vi "Teleop.vi"(10 "Match Info":T1={"Autonomous Elapsed Seconds"=0.0, "TeleOp Elapsed Seconds"=0.0, "Disabled Elapsed Seconds"=0.0, "Visited Autonomous"=FALSE, "Visited TeleOp"=FALSE, "Visited Disabled"=FALSE, "Autonomous Settings"={"Autonomous Style"=enum."Independent", "VI Refnum"=refnum}}, 11 "Call Context":T2) -> ()   [LabVIEW 2013]
doc: "This VI is called for each TeleOp packet received from the DS where the robot is not disabled. It is often used to read from the joysticks and update I/O or to update setpoints for timed control loops. It should complete and return within 20 milliseconds or it may miss DS packets."
uses:
  <vilib>/Rock Robotics/WPI/DriverStation/WPI_DriverStationDerivedRobotMode.ctl
  <vilib>/Rock Robotics/WPI/DriverStation/WPI_DriverStationMatch Info.ctl
  <vilib>/Rock Robotics/WPI/Solenoid/WPI_SolenoidValue.ctl
  Robot Global Data.vi
  <vilib>/Rock Robotics/WPI/Joystick/WPI_JoystickGetSetRefNum.vi
  <vilib>/Rock Robotics/WPI/Solenoid/Deprecated/WPI_SolenoidGetBool.vi
  <vilib>/Rock Robotics/WPI/Solenoid/WPI_SolenoidSetEnum.vi
  <vilib>/Rock Robotics/WPI/RobotDrive/WPI_RobotDriveGetSetRefNum.vi
  Labview/Sub VIs/Sting Pot Value.vi
panel:
  out "Voltage":dbl
  out "Value":bool
  out "Numeric 1":dbl(slide) scale=0.0..100.0
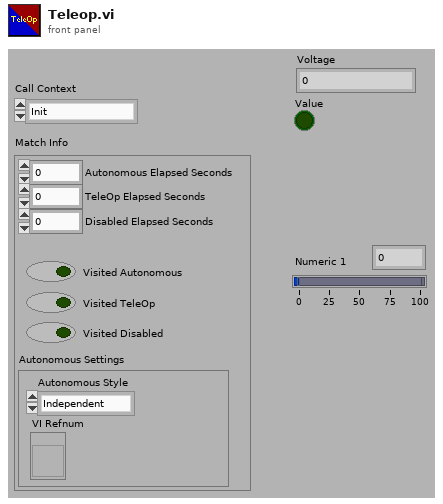
[diagram p1: front panel]
types:
  T1 = typedef "WPI_DriverStationMatch Info.ctl" = cluster{"Autonomous Elapsed Seconds":dbl, "TeleOp Elapsed Seconds":dbl, "Disabled Elapsed Seconds":dbl, "Visited Autonomous":bool, "Visited TeleOp":bool, "Visited Disabled":bool, "Autonomous Settings":cluster{"Autonomous Style":enum16{"Iterative", "Independent"}, "VI Refnum":refnum<vi>}}
  T2 = typedef "WPI_DriverStationDerivedRobotMode.ctl" = enum16{"Init", "Execute", "Stop"}
  T3 = typedef "WPI_JoystickDevRef.ctl" = cluster{"Device":T4}
  T4 = typedef "WPI_JoystickDeviceEnum.ctl" = enum16{"USB 1", "USB 2", "USB 3", "USB 4", "Kinect 1", "Kinect 2"}
  T5 = typedef "WPI_JoystickButtonState.ctl" = cluster{"Button 1":bool, "Button 2":bool, "Button 3":bool, "Button 4":bool, "Button 5":bool, "Button 6":bool, "Button 7":bool, "Button 8":bool, "Button 9":bool, "Button 10":bool, "Button 11":bool, "Button 12":bool}
  T6 = typedef "WPI_MotorControlDeviceRef.ctl" = cluster{"DeviceStatus":errorcluster, "Type":enum16{"PWM", "CAN"}, "PWM":cluster{"Digital Module":T7, "PWM Channel":T8, "DeadBand":T9}, "CAN":cluster{"Device Number":u8, "Control Mode":T10, "Semaphore":T11, "Max Vout":dbl}, "Invert":bool, "TransformRef":T12, "InvTransformRef":T12}
  T7 = typedef "FPGA_TypedefDigitalModule.ctl" = enum16{"Digital Module 1", "Digital Module 2"}
  T8 = typedef "FPGA_DIOPWMChannel.ctl" = enum8{"PWM 1", "PWM 2", "PWM 3", "PWM 4", "PWM 5", "PWM 6", "PWM 7", "PWM 8", "PWM 9", "PWM 10", "Invalid"}
  T9 = typedef "WPI_PWMDeadband.ctl" = cluster{"Name":string, "maxPositivePwm":i32, "minPositivePwm":i32, "centerPwm":i32, "maxNegativePwm":i32, "minNegativePwm":i32, "angularRange":u16}
  T10 = typedef "WPI_CANJaguar_ControlMode.ctl" = enum8{"Percent VBus", "Current", "Speed", "Position", "Voltage"}
  T11 = typedef "Semaphore RefNum" = refnum<k1>
  T12 = typedef "WPI_PWMTransform_ConPane.ctl" = refnum<vi>
  T13 = typedef "WPI_AnalogChannelDevRef.ctl" = cluster{"DevStatus":errorcluster, "Analog Module":T14, "Analog Channel":T15}
  T14 = typedef "FPGA_TypedefAnalogModule.ctl" = enum16{"Analog Module 1", "Analog Module 2"}
  T15 = typedef "FPGA_AIChannel.ctl" = enum8{"AI 1", "AI 2", "AI 3", "AI 4", "AI 5", "AI 6", "AI 7", "AI 8", "Invalid"}
  T16 = cluster{"axis 1 (x)":dbl, "axis 2 (y)":dbl, "axis 3 (throttle)":dbl, "axis 4":dbl, "axis 5":dbl, "axis 6":dbl}
  T17 = typedef "WPI_RobotDriveDevRef.ctl" = cluster{"DevStatus":errorcluster, "Motors[]":T6[], "Square Inputs":bool, "Max Output":dbl, "Isochronous":bool}
  T18 = typedef "WPI_RelayDevRef.ctl" = cluster{"DevStatus":errorcluster, "Relay Channel":T19, "Digital Module":T7, "Relay Direction":T20}
  T19 = typedef "FPGA_DIORelayChannel.ctl" = enum8{"Relay 1", "Relay 2", "Relay 3", "Relay 4", "Relay 5", "Relay 6", "Relay 7", "Relay 8", "Invalid"}
  T20 = typedef "WPI_RelayDirection.ctl" = enum16{"Both directions", "Forward only", "Reverse only"}
  T21 = typedef "WPI_DigitalInputDevRef.ctl" = cluster{"DevStatus":errorcluster, "DIO Channel":T22, "Digital Module":T7}
  T22 = typedef "FPGA_DIOChannel.ctl" = enum8{"DIO 1", "DIO 2", "DIO 3", "DIO 4", "DIO 5", "DIO 6", "DIO 7", "DIO 8", "DIO 9", "DIO 10", "DIO 11", "DIO 12", "DIO 13", "DIO 14", "Invalid"}
  T23 = typedef "WPI_SolenoidValue.ctl" = enum16{"Off", "On", "Forward", "Reverse"}
  T24 = typedef "WPI_SolenoidDevRef.ctl" = cluster{"DevStatus":errorcluster, "Solenoid Module":T25, "Forward Solenoid Channel":T26, "Reverse Solenoid Channel":T26}
  T25 = typedef "FPGA_TypedefSolenoidModule.ctl" = enum16{"Solenoid Module 1", "Solenoid Module 2"}
  T26 = typedef "WPI_SolenoidChannel.ctl" = enum8{"Solenoid 1", "Solenoid 2", "Solenoid 3", "Solenoid 4", "Solenoid 5", "Solenoid 6", "Solenoid 7", "Solenoid 8", "Invalid"}
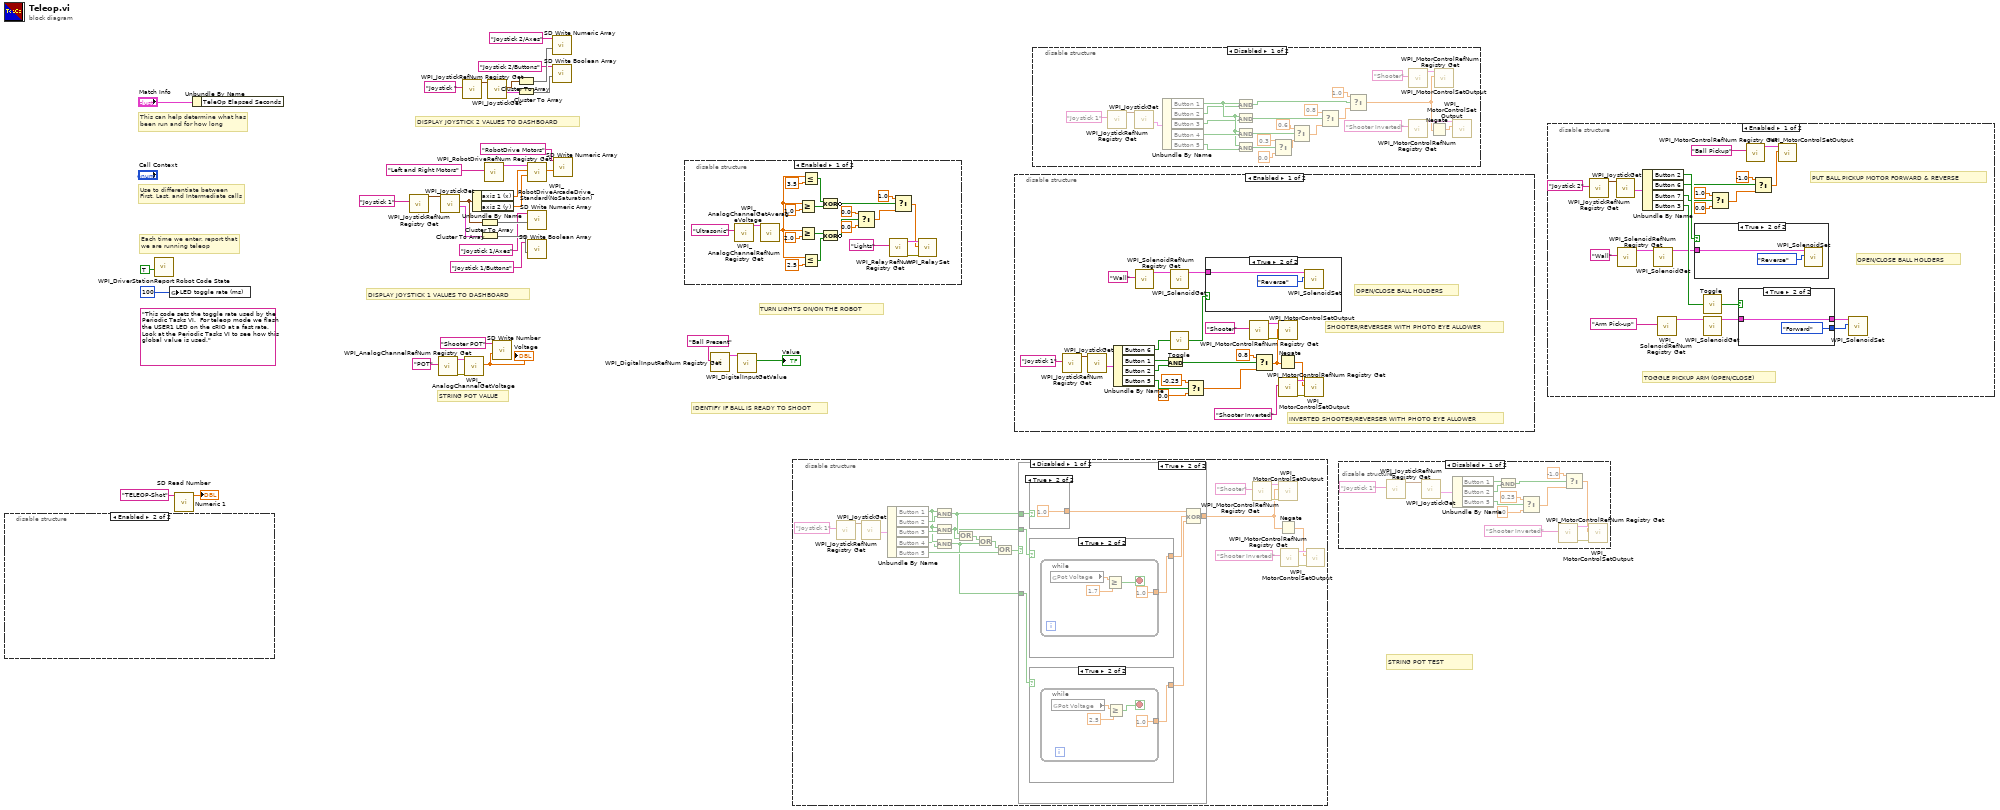
[diagram p0: block diagram]
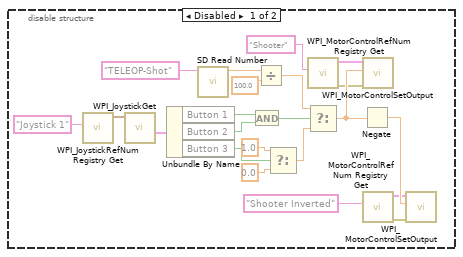
[diagram p2: hidden frame]
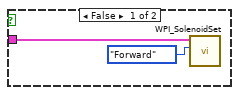
[diagram p3: hidden frame]
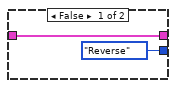
[diagram p4: hidden frame]
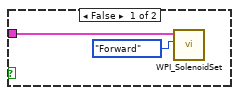
[diagram p6: hidden frame]
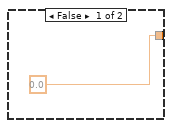
[diagram p9: hidden frame]
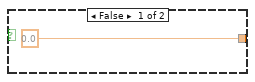
[diagram p10: hidden frame]
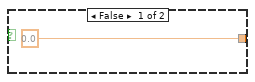
[diagram p11: hidden frame]
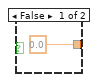
[diagram p12: hidden frame]
diagram:
  (unwired) "This code sets the toggle rate used by the Periodic Tasks VI.  For teleop mode we flash the USER1 LED on the cRIO at a fast rate.  Look at the Periodic Tasks VI to see how this global value is used."
  # "STRING POT TEST"
  # "DISPLAY JOYSTICK 1 VALUES TO DASHBOARD"
  # "DISPLAY JOYSTICK 2 VALUES TO DASHBOARD"
  # "IDENTIFY IF BALL IS READY TO SHOOT"
  # "TURN LIGHTS ON/ON THE ROBOT"
  # "STRING POT VALUE"
  # "Each time we enter, report that\nwe are running teleop"
  # "Use to differentiate between\nFirst, Last, and Intermediate calls"
  # "This can help determine what has\nbeen run and for how long"
  n1 = disable-structure shown="Enabled" {
    frame Disabled {
      n2 = call <vilib>:"WPI_JoystickRefNum Registry Get.vi"("refnum name"="Joystick 1") -> ("JoystickDevRef"=w37:T3)  [unwired: 9 in, 1 out]
      n3 = call <vilib>:"WPI_JoystickGet.vi"("JoystickDevRef"=w37) -> ("Buttons"=w38:T5)  [unwired: 4 in, 2 out]
      n4 = Unbundle By Name(w38) -> ("Button 1"=w40:bool, "Button 2"=w39:bool, "Button 3"=w43:bool)
      n5 = call <vilib>:"SD Read Number.vi"("Name"="TELEOP-Shot" ("refnum name")) -> ("Numeric"=w56:dbl)  [unwired: 8 in, 2 out]
      n6 = And(x=w40, y=w39) -> (x .and. y?=w41:bool)
      n7 = Divide(x=w56, y=100.0) -> (x/y=w57:dbl)
      n8 = Select(t=1.0, s=w43, f=0.0) -> (s? t:f=w46:dbl)
      n9 = call <vilib>:"WPI_MotorControlRefNum Registry Get.vi"("refnum name"="Shooter") -> ("error out"=w47:errorcluster, "MotorControlDevRef"=w48:T6)  [unwired: 9 in]
      n10 = Select(t=w57, s=w41, f=w46) -> (s? t:f=w52:dbl)
      n11 = Negate(x=w52) -> (-x=w53:dbl)
      n12 = call <vilib>:"WPI_MotorControlSetOutput.vi"("error in (no error)"=w47, "Output"=w52, "MotorControlDevRef"=w48) -> ()  [unwired: 6 in, 3 out]
      n13 = call <vilib>:"WPI_MotorControlRefNum Registry Get.vi"("refnum name"="Shooter Inverted") -> ("error out"=w50:errorcluster, "MotorControlDevRef"=w51:T6)  [unwired: 9 in]
      n14 = call <vilib>:"WPI_MotorControlSetOutput.vi"("error in (no error)"=w50, "Output"=w53, "MotorControlDevRef"=w51) -> ()  [unwired: 6 in, 3 out]
    }
    frame Enabled {
    }
  }
  n15 = call <vilib>:"WPI_DriverStationReport Robot Code State.vi"("TeleOp"=TRUE ("Autonomous")) -> ()  [unwired: 10 in, 1 out]
  n16 = global write "Robot Global Data.vi" "LED toggle rate (ms)"(u32 100 ("LED ms toggle rate")) -> ()
  n17 = call <vilib>:"SD Read Number.vi"("Name"="TELEOP-Shot" ("refnum name")) -> ("Numeric"=→"Numeric 1":dbl)  [unwired: 8 in, 2 out]
  n18 = Unbundle By Name("Match Info") -> ()  [unwired: 1 out]
  n19 = call <vilib>:"WPI_JoystickRefNum Registry Get.vi"("refnum name"="Joystick 1") -> ("JoystickDevRef"=w29:T3)  [unwired: 1 in, 9 out]
  n20 = call <vilib>:"WPI_AnalogChannelRefNum Registry Get.vi"("refnum name"="POT") -> ("error out"=w15:errorcluster, "AIDeviceRef"=w16:T13)  [unwired: 9 in]
  n21 = call <vilib>:"WPI_JoystickGet.vi"("JoystickDevRef"=w29) -> ("Buttons"=w26:T5, "Axes"=w23:T16)  [unwired: 1 in, 4 out]
  n22 = call <vilib>:"WPI_JoystickRefNum Registry Get.vi"("refnum name"="Joystick ") -> ("JoystickDevRef"=w5:T3)  [unwired: 1 in, 9 out]
  n23 = call <vilib>:"WPI_AnalogChannelGetVoltage.vi"("error in (no error)"=w15, "AIDeviceRef"=w16) -> ("Voltage"=w13:dbl)  [unwired: 7 in, 2 out]
  "Voltage" <- w13
  n24 = Unbundle By Name(w23) -> ("axis 1 (x)"=w32:dbl, "axis 2 (y)"=w31:dbl)
  n25 = Cluster To Array(cluster=w23) -> (array=w22:dbl[])
  n26 = Cluster To Array(cluster=w26) -> (array=w25:bool[])
  n27 = call <vilib>:"WPI_RobotDriveRefNum Registry Get.vi"("refnum name"="Left and Right Motors") -> ("RobotDriveDevRef"=w33:T17)  [unwired: 1 in, 9 out]
  n28 = call <vilib>:"WPI_JoystickGet.vi"("JoystickDevRef"=w5) -> ("Buttons"=w6:T5, "Axes"=w9:T16)  [unwired: 1 in, 4 out]
  n29 = call <vilib>:"SD Write Number.vi"("Numeric"=w13, "Name"="Shooter POT" ("Table Prefix out")) -> ()  [unwired: 8 in, 2 out]
  n30 = Cluster To Array(cluster=w9) -> (array=w10:dbl[])
  n31 = Cluster To Array(cluster=w6) -> (array=w7:bool[])
  n32 = call <vilib>:"WPI_RobotDriveArcadeDrive_Standard(NoSaturation).vi"("Y axis value"=w31, "X axis value"=w32, "RobotDriveDevRef"=w33) -> ("Motor Values"=w19:dbl[])  [unwired: 1 in, 7 out]
  n33 = call <vilib>:"SD Write Numeric Array.vi"("Numeric Array"=w22, "Name"="Joystick 1/Axes") -> ()  [unwired: 8 in, 2 out]
  n34 = call <vilib>:"SD Write Boolean Array.vi"("Boolean Array"=w25, "Name"="Joystick 1/Buttons") -> ()  [unwired: 8 in, 2 out]
  n35 = call <vilib>:"SD Write Numeric Array.vi"("Numeric Array"=w10, "Name"="Joystick 2/Axes") -> ()  [unwired: 8 in, 2 out]
  n36 = call <vilib>:"SD Write Boolean Array.vi"("Boolean Array"=w7, "Name"="Joystick 2/Buttons") -> ()  [unwired: 8 in, 2 out]
  n37 = call <vilib>:"SD Write Numeric Array.vi"("Numeric Array"=w19, "Name"="RobotDrive Motors") -> ()  [unwired: 8 in, 2 out]
  n38 = disable-structure shown="Enabled" {
    frame Enabled {
      n39 = call <vilib>:"WPI_AnalogChannelRefNum Registry Get.vi"("refnum name"="Ultrasonic") -> ("AIDeviceRef"=w77:T13)  [unwired: 9 in, 1 out]
      n40 = call <vilib>:"WPI_AnalogChannelGetAverageVoltage.vi"("AIDeviceRef"=w77) -> ("Voltage"=w68:dbl)  [unwired: 8 in, 2 out]
      n41 = Greater Or Equal?(x=w68, y=1.0) -> (x >= y?=w71:bool)
      n42 = Greater Or Equal?(x=w68, y=2.0) -> (x >= y?=w65:bool)
      n43 = Less Or Equal?(x=w68, y=3.5) -> (x <= y?=w70:bool)
      n44 = Less Or Equal?(x=w68, y=2.5) -> (x <= y?=w66:bool)
      n45 = Compound Arithmetic op=XOR(w70, w71) -> (invert w63:bool)
      n46 = Compound Arithmetic op=XOR(w65, w66) -> (invert w64:bool)
      n47 = Select(t=0.0, s=w64, f=0.0) -> (s? t:f=w59:dbl)
      n48 = call <vilib>:"WPI_RelayRefNum Registry Get.vi"("refnum name"="Lights") -> ("error out"=w76:errorcluster, "RelayDevRef"=w75:T18)  [unwired: 9 in]
      n49 = Select(t=1.0, s=w63, f=w59) -> (s? t:f=w58:dbl)
      n50 = call <vilib>:"WPI_RelaySet.vi"("error in (no error)"=w76, "RelayValue"=w58, "RelayDevRef"=w75) -> ()  [unwired: 7 in, 2 out]
    }
    frame Disabled {
    }
  }
  n51 = call <vilib>:"WPI_DigitalInputRefNum Registry Get.vi"("refnum name"="Ball Present") -> ("DigitalInputDevRef"=w2:T21)  [unwired: 9 in, 1 out]
  n52 = call <vilib>:"WPI_DigitalInputGetValue.vi"("DigitalInputDevRef"=w2) -> ("Value"=→"Value":bool)  [unwired: 8 in, 2 out]
  n53 = disable-structure shown="Disabled" {
    frame Disabled {
      n54 = call <vilib>:"WPI_JoystickRefNum Registry Get.vi"("refnum name"="Joystick 1") -> ("JoystickDevRef"=w99:T3)  [unwired: 9 in, 1 out]
      n55 = call <vilib>:"WPI_JoystickGet.vi"("JoystickDevRef"=w99) -> ("Buttons"=w100:T5)  [unwired: 4 in, 2 out]
      n56 = Unbundle By Name(w100) -> ("Button 1"=w95:bool, "Button 2"=w97:bool, "Button 3"=w96:bool, "Button 4"=w94:bool, "Button 5"=w91:bool)
      n57 = And(x=w95, y=w97) -> (x .and. y?=w89:bool)
      n58 = And(x=w95, y=w96) -> (x .and. y?=w88:bool)
      n59 = And(x=w95, y=w94) -> (x .and. y?=w79:bool)
      n60 = Or(x=w89, y=w88) -> (x .or. y?=w93:bool)
      n61 = Or(x=w93, y=w79) -> (x .or. y?=w92:bool)
      n62 = Or(x=w92, y=w91) -> (x .or. y?=w90:bool)
      n63 = case shown="True" w90 {
        tunnel: w89 -> [_ w108]
        tunnel: w88 -> [_ w107]
        tunnel: [0.0 w103] -> w81
        tunnel: w79 -> [_ w102]
        frame False {
        }
        frame True {
          n64 = case shown="True" w108 {
            tunnel: [0.0 1.0] -> w106
            frame False {
            }
            frame True {
            }
          }
          n65 = case shown="True" w107 {
            tunnel: [0.0 w116] -> w105
            frame False {
            }
            frame True {
              n66 = while {
                tunnel: [1.0] -> w116
                stop <- w119 stop-if-true
                n67 = global read "Sting Pot Value.vi" "Pot Voltage"() -> (w118:dbl)
                n68 = Greater Or Equal?(x=w118, y=1.7) -> (x >= y?=w119:bool)
              }
            }
          }
          n69 = case shown="True" w102 {
            tunnel: [0.0 w110] -> w104
            frame False {
            }
            frame True {
              n70 = while {
                tunnel: [1.0] -> w110
                stop <- w111 stop-if-true
                n71 = global read "Sting Pot Value.vi" "Pot Voltage"() -> (w112:dbl)
                n72 = Greater Or Equal?(x=w112, y=2.5) -> (x >= y?=w111:bool)
              }
            }
          }
          n73 = Compound Arithmetic op=XOR(w106, w105, w104) -> (w103:i32)
        }
      }
      n74 = call <vilib>:"WPI_MotorControlRefNum Registry Get.vi"("refnum name"="Shooter") -> ("error out"=w83:errorcluster, "MotorControlDevRef"=w82:T6)  [unwired: 9 in]
      n75 = call <vilib>:"WPI_MotorControlSetOutput.vi"("error in (no error)"=w83, "Output"=w81, "MotorControlDevRef"=w82) -> ()  [unwired: 6 in, 3 out]
      n76 = Negate(x=w81) -> (-x=w80:dbl)
      n77 = call <vilib>:"WPI_MotorControlRefNum Registry Get.vi"("refnum name"="Shooter Inverted") -> ("error out"=w86:errorcluster, "MotorControlDevRef"=w87:T6)  [unwired: 9 in]
      n78 = call <vilib>:"WPI_MotorControlSetOutput.vi"("error in (no error)"=w86, "Output"=w80, "MotorControlDevRef"=w87) -> ()  [unwired: 6 in, 3 out]
    }
    frame Enabled {
    }
  }
  n79 = disable-structure shown="Enabled" {
    frame Enabled {
      # "OPEN/CLOSE BALL HOLDERS"
      # "SHOOTER/REVERSER WITH PHOTO EYE ALLOWER"
      # "INVERTED SHOOTER/REVERSER WITH PHOTO EYE ALLOWER"
      n80 = call <vilib>:"WPI_JoystickRefNum Registry Get.vi"("refnum name"="Joystick 1") -> ("JoystickDevRef"=w142:T3)  [unwired: 9 in, 1 out]
      n81 = call <vilib>:"WPI_JoystickGet.vi"("JoystickDevRef"=w142) -> ("Buttons"=w141:T5)  [unwired: 4 in, 2 out]
      n82 = Unbundle By Name(w141) -> ("Button 6"=w124:bool, "Button 1"=w137:bool, "Button 2"=w125:bool, "Button 5"=w136:bool)
      n83 = call <vilib>:"WPI_SolenoidRefNum Registry Get.vi"("refnum name"="Wall") -> ("SolenoidDevRef"=w145:T24)  [unwired: 9 in, 1 out]
      n84 = And(x=w137, y=w125) -> (x .and. y?=w131:bool)
      n85 = call-poly <vilib>:"WPI_SolenoidGet.vi"("SolenoidDevRef"=w145) -> ("SolenoidDevRef"=w146:T24)  [unwired: 8 in, 2 out]
      n86 = call "Toggle.vi"("Input"=w124) -> ("Toggled Output"=w123:bool)
      n87 = Select(t=-0.25, s=w136, f=0.0) -> (s? t:f=w134:dbl)
      n88 = case shown="True" w123 {
        tunnel: w146 -> [w148 w150]
        frame False {
          n89 = call-poly <vilib>:"WPI_SolenoidSet.vi"("Value"=WPI_SolenoidValue."Forward", "SolenoidDevRef"=w148) -> ()  [unwired: 8 in, 2 out]
        }
        frame True {
          n90 = call-poly <vilib>:"WPI_SolenoidSet.vi"("Value"=WPI_SolenoidValue."Reverse", "SolenoidDevRef"=w150) -> ()  [unwired: 8 in, 2 out]
        }
      }
      n91 = call <vilib>:"WPI_MotorControlRefNum Registry Get.vi"("refnum name"="Shooter") -> ("error out"=w139:errorcluster, "MotorControlDevRef"=w138:T6)  [unwired: 9 in]
      n92 = Select(t=0.8, s=w131, f=w134) -> (s? t:f=w127:dbl)
      n93 = Negate(x=w127) -> (-x=w126:dbl)
      n94 = call <vilib>:"WPI_MotorControlSetOutput.vi"("error in (no error)"=w139, "Output"=w127, "MotorControlDevRef"=w138) -> ()  [unwired: 6 in, 3 out]
      n95 = call <vilib>:"WPI_MotorControlRefNum Registry Get.vi"("refnum name"="Shooter Inverted") -> ("error out"=w129:errorcluster, "MotorControlDevRef"=w128:T6)  [unwired: 9 in]
      n96 = call <vilib>:"WPI_MotorControlSetOutput.vi"("error in (no error)"=w129, "Output"=w126, "MotorControlDevRef"=w128) -> ()  [unwired: 6 in, 3 out]
    }
    frame Disabled {
    }
  }
  n97 = disable-structure shown="Disabled" {
    frame Disabled {
      n98 = call <vilib>:"WPI_JoystickRefNum Registry Get.vi"("refnum name"="Joystick 1") -> ("JoystickDevRef"=w153:T3)  [unwired: 9 in, 1 out]
      n99 = call <vilib>:"WPI_JoystickGet.vi"("JoystickDevRef"=w153) -> ("Buttons"=w151:T5)  [unwired: 4 in, 2 out]
      n100 = Unbundle By Name(w151) -> ("Button 1"=w156:bool, "Button 2"=w154:bool, "Button 3"=w155:bool, "Button 4"=w157:bool, "Button 5"=w158:bool)
      n101 = And(x=w156, y=w154) -> (x .and. y?=w159:bool)
      n102 = And(x=w156, y=w155) -> (x .and. y?=w165:bool)
      n103 = And(x=w156, y=w157) -> (x .and. y?=w164:bool)
      n104 = And(x=w156, y=w158) -> (x .and. y?=w163:bool)
      n105 = Select(t=0.3, s=w163, f=0.0) -> (s? t:f=w162:dbl)
      n106 = Select(t=0.6, s=w164, f=w162) -> (s? t:f=w161:dbl)
      n107 = Select(t=0.8, s=w165, f=w161) -> (s? t:f=w160:dbl)
      n108 = Select(t=1.0, s=w159, f=w160) -> (s? t:f=w174:dbl)
      n109 = call <vilib>:"WPI_MotorControlRefNum Registry Get.vi"("refnum name"="Shooter Inverted") -> ("MotorControlDevRef"=w175:T6)  [unwired: 9 in, 1 out]
      n110 = call <vilib>:"WPI_MotorControlRefNum Registry Get.vi"("refnum name"="Shooter") -> ("MotorControlDevRef"=w172:T6)  [unwired: 9 in, 1 out]
      n111 = Negate(x=w174) -> (-x=w173:dbl)
      n112 = call <vilib>:"WPI_MotorControlSetOutput.vi"("Output"=w174, "MotorControlDevRef"=w172) -> ()  [unwired: 7 in, 3 out]
      n113 = call <vilib>:"WPI_MotorControlSetOutput.vi"("Output"=w173, "MotorControlDevRef"=w175) -> ()  [unwired: 7 in, 3 out]
    }
    frame Enabled {
    }
  }
  n114 = disable-structure shown="Disabled" {
    frame Disabled {
      n115 = call <vilib>:"WPI_JoystickRefNum Registry Get.vi"("refnum name"="Joystick 1") -> ("JoystickDevRef"=w190:T3)  [unwired: 9 in, 1 out]
      n116 = call <vilib>:"WPI_JoystickGet.vi"("JoystickDevRef"=w190) -> ("Buttons"=w191:T5)  [unwired: 4 in, 2 out]
      n117 = Unbundle By Name(w191) -> ("Button 1"=w187:bool, "Button 2"=w188:bool, "Button 5"=w183:bool)
      n118 = And(x=w187, y=w188) -> (x .and. y?=w177:bool)
      n119 = Select(t=0.25, s=w183, f=0.0) -> (s? t:f=w182:dbl)
      n120 = call <vilib>:"WPI_MotorControlRefNum Registry Get.vi"("refnum name"="Shooter Inverted") -> ("error out"=w185:errorcluster, "MotorControlDevRef"=w186:T6)  [unwired: 9 in]
      n121 = Select(t=-1.0, s=w177, f=w182) -> (s? t:f=w178:dbl)
      n122 = call <vilib>:"WPI_MotorControlSetOutput.vi"("error in (no error)"=w185, "Output"=w178, "MotorControlDevRef"=w186) -> ()  [unwired: 6 in, 3 out]
    }
    frame Enabled {
    }
  }
  n123 = disable-structure shown="Enabled" {
    frame Enabled {
      # "OPEN/CLOSE BALL HOLDERS"
      # "TOGGLE PICKUP ARM (OPEN/CLOSE)"
      # "PUT BALL PICKUP MOTOR FORWARD & REVERSE"
      n124 = call <vilib>:"WPI_JoystickRefNum Registry Get.vi"("refnum name"="Joystick 2") -> ("JoystickDevRef"=w212:T3)  [unwired: 9 in, 1 out]
      n125 = call <vilib>:"WPI_JoystickGet.vi"("JoystickDevRef"=w212) -> ("Buttons"=w211:T5)  [unwired: 4 in, 2 out]
      n126 = call <vilib>:"WPI_SolenoidRefNum Registry Get.vi"("refnum name"="Wall") -> ("SolenoidDevRef"=w203:T24)  [unwired: 9 in, 1 out]
      n127 = Unbundle By Name(w211) -> ("Button 2"=w201:bool, "Button 6"=w193:bool, "Button 7"=w192:bool, "Button 3"=w205:bool)
      n128 = call-poly <vilib>:"WPI_SolenoidGet.vi"("SolenoidDevRef"=w203) -> ("SolenoidDevRef"=w202:T24)  [unwired: 8 in, 2 out]
      n129 = call <vilib>:"WPI_SolenoidRefNum Registry Get.vi"("refnum name"="Arm Pick-up") -> ("SolenoidDevRef"=w210:T24)  [unwired: 9 in, 1 out]
      n130 = case shown="True" w201 {
        tunnel: w202 -> [w216 w218]
        frame False {
          n131 = call-poly <vilib>:"WPI_SolenoidSet.vi"("Value"=WPI_SolenoidValue."Forward", "SolenoidDevRef"=w216) -> ()  [unwired: 8 in, 2 out]
        }
        frame True {
          n132 = call-poly <vilib>:"WPI_SolenoidSet.vi"("Value"=WPI_SolenoidValue."Reverse", "SolenoidDevRef"=w218) -> ()  [unwired: 8 in, 2 out]
        }
      }
      n133 = call "Toggle.vi"("Input"=w205) -> ("Toggled Output"=w209:bool)
      n134 = call-poly <vilib>:"WPI_SolenoidGet.vi"("SolenoidDevRef"=w210) -> ("SolenoidDevRef"=w208:T24)  [unwired: 8 in, 2 out]
      n135 = Select(t=1.0, s=w192, f=0.0) -> (s? t:f=w199:dbl)
      n136 = case shown="True" w209 {
        tunnel: w208 -> [w220 w222]
        tunnel: [w220 w222] -> w207
        tunnel: [WPI_SolenoidValue."Reverse" ("Value") WPI_SolenoidValue."Forward" ("Value")] -> w206
        frame False {
        }
        frame True {
        }
      }
      n137 = call <vilib>:"WPI_MotorControlRefNum Registry Get.vi"("refnum name"="Ball Pickup") -> ("MotorControlDevRef"=w195:T6)  [unwired: 9 in, 1 out]
      n138 = Select(t=-1.0, s=w193, f=w199) -> (s? t:f=w200:dbl)
      n139 = call <vilib>:"WPI_MotorControlSetOutput.vi"("Output"=w200, "MotorControlDevRef"=w195) -> ()  [unwired: 7 in, 3 out]
      n140 = call-poly <vilib>:"WPI_SolenoidSet.vi"("Value"=w206, "SolenoidDevRef"=w207) -> ()  [unwired: 8 in, 2 out]
    }
    frame Disabled {
    }
  }
